vi "Two Button Dialog_TouchScreen.vi"(1 "F button name (\"Cancel\")":string, 2 "T button name (\"OK\")":string, 3 "Message":string) -> (0 "T Button?":T1)   [LabVIEW 2010]
uses:
  _TypeDefs/OK Button_TouchScreen.ctl
panel:
  in  "F Button":T1
  in  "T Button":T1
  out "Message Indicator":string
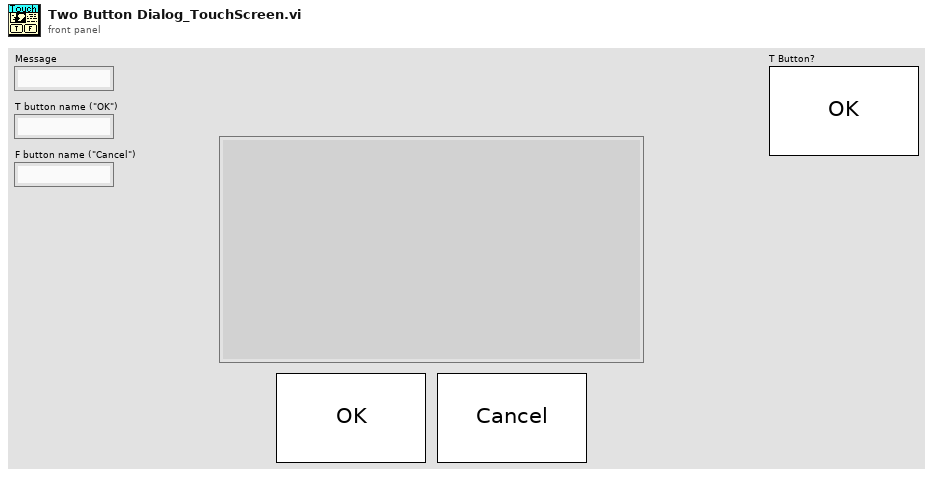
[diagram p1: front panel]
types:
  T1 = typedef "OK Button_TouchScreen.ctl" = bool
  T2 = enum8{"Enabled", "Disabled", "Disabled and Grayed Out"}
  T3 = cluster{"left":i16, "top":i16, "right":i16, "bottom":i16}
  T4 = typedef "LVBoundsTypeDef.ctl" = cluster{"Width":u32, "Height":u32}
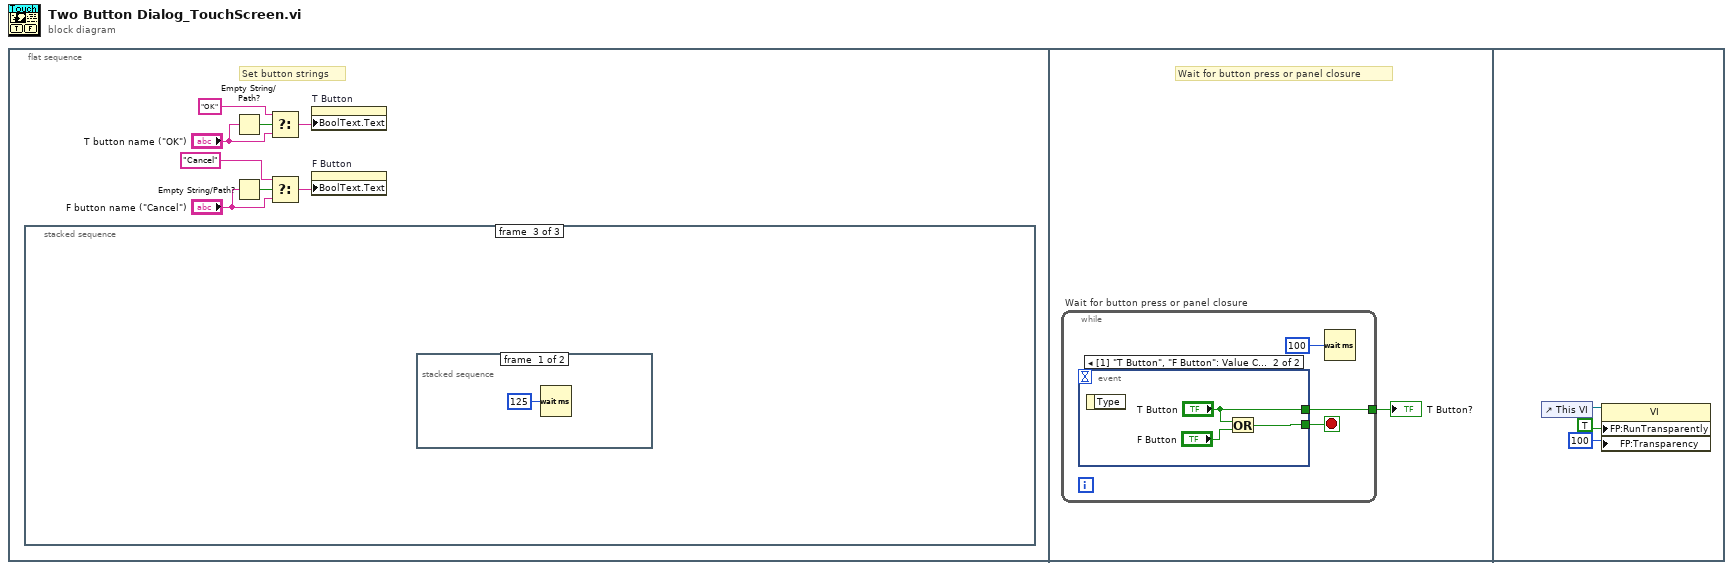
[diagram p0: block diagram]
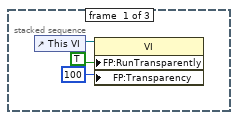
[diagram p2: hidden frame]
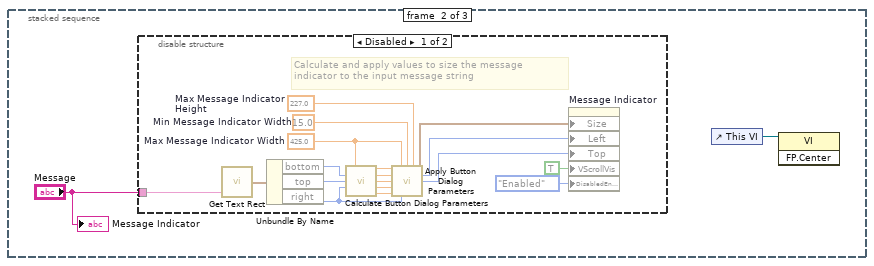
[diagram p3: hidden frame]
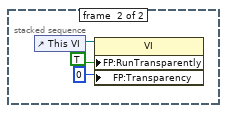
[diagram p5: hidden frame]
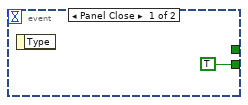
[diagram p6: hidden frame]
diagram:
  n1 = flat-sequence {
    frame #0 {
      # "Set button strings"
      n2 = stacked-sequence {
        frame #0 {
          n3 = control-ref of="This VI"() -> (w9:refnum<vi>)
          n4 = property class="VI"(reference=w9, "FP:RunTransparently"=TRUE, "FP:Transparency"=u8 100 ("Front Panel Window:Transparency")) -> ()  [unwired: 1 in, 2 out]
        }
        frame #1 {
          n5 = disable-structure shown="Disabled" {
            disable-tunnel: "Message" -> [w31 _]
            frame Disabled {
              w22 = 15.0  # Min Message Indicator Width
              w21 = 227.0  # Max Message Indicator Height
              w25 = 425.0  # Max Message Indicator Width
              # "Calculate and apply values to size the message indicator to the input message string"
              n6 = call <vilib>:"Get Text Rect.vi"("text"=w31) -> ("rect"=w29:T3)  [unwired: 8 in]
              n7 = Unbundle By Name(w29) -> ("bottom"=w17:i16, "top"=w18:i16, "right"=w16:i16)
              n8 = call "Calculate Button Dialog Parameters.vi"("Max Message Indicator Width"=w25, "bottom"=w17, "top"=w18, "right"=w16) -> ("Indicator left position"=w26:dbl, "Calculated indicator height"=w24:dbl, "Indicator height scaled large"=w23:dbl, "Actual indicator height"=w20:dbl, "Indicator height scaled small"=w19:dbl)  [unwired: 7 in]
              n9 = call "Apply Button Dialog Parameters.vi"("Indicator left position"=w26, "Max Message Indicator Width"=w25, "Min Message Indicator Width"=w22, "Max Message Indicator Height"=w21, "Calculated indicator height"=w24, "Indicator height scaled large"=w23, "Actual indicator height"=w20, "Indicator height scaled small"=w19, "right"=w16) -> ("Message indicator size"=w30:T4, "Message indicator left"=w28:i32, "Message indicator top"=w27:i32)  [unwired: 1 in, 3 out]
              n10 = property on="Message Indicator" class="Str"("Size"=w30, "Left"=w28, "Top"=w27, "VScrollVis"=TRUE ("Vertical Scrollbar Visible"), "DisabledEnum"=T2."Enabled" ("Disabled")) -> ()  [unwired: 2 in, 2 out]
            }
            frame Enabled {
            }
          }
          n11 = control-ref of="This VI"() -> (w12:refnum<vi>)
          n12 = invoke class="VI" method="FP.Center"(reference=w12) -> ()  [unwired: 2 in, 3 out]
          "Message Indicator" <- "Message"
        }
        frame #2 {
          n13 = stacked-sequence {
            frame #0 {
              n14 = Wait (ms)(milliseconds to wait=u32 125) -> ()  [unwired: 1 out]
            }
            frame #1 {
              n15 = control-ref of="This VI"() -> (w35:refnum<vi>)
              n16 = property class="VI"(reference=w35, "FP:RunTransparently"=TRUE, "FP:Transparency"=u8 0 ("Front Panel Window:Transparency")) -> ()  [unwired: 1 in, 2 out]
            }
          }
        }
      }
      n17 = Empty String/Path?(string/path="T button name (\"OK\")") -> (empty?=w7:bool)
      n18 = Empty String/Path?(string/path="F button name (\"Cancel\")") -> (empty?=w2:bool)
      n19 = Select(t="OK", s=w7, f="T button name (\"OK\")") -> (s? t:f=w5:string)
      n20 = Select(t="Cancel", s=w2, f="F button name (\"Cancel\")") -> (s? t:f=w1:string)
      n21 = property on="T Button" class="Bool"("BoolText.Text"=w5) -> ()  [unwired: 2 in, 2 out]
      n22 = property on="F Button" class="Bool"("BoolText.Text"=w1) -> ()  [unwired: 2 in, 2 out]
    }
    frame #1 {
      # "Wait for button press or panel closure"
      n23 = while "Wait for button press or panel closure" {
        tunnel: [w37] -> w36
        stop <- w38 stop-if-true
        n24 = event shown="[1] \"T Button\", \"F Button\": Value Change" {
          selector: _ -> [_ _]
          dyn-events: _ -> [_ _]
          timeout: _ -> [_ _]
          tunnel: [T1 TRUE ("T Button") w42] -> w38
          tunnel: [_ "T Button"] -> w37
          event Panel Close {
            n25 = event-data() -> ()  [unwired: 1 in, 1 out]
          }
          event Value Change {
            n26 = event-data() -> ()  [unwired: 1 in, 1 out]
            n27 = Or(x="T Button", y="F Button") -> (x .or. y?=w42:T1)
          }
        }
        n28 = Wait (ms)(milliseconds to wait=u32 100) -> ()  [unwired: 1 out]
      }
      "T Button?" <- w36
    }
    frame #2 {
      n29 = control-ref of="This VI"() -> (w46:refnum<vi>)
      n30 = property class="VI"(reference=w46, "FP:RunTransparently"=TRUE, "FP:Transparency"=u8 100 ("Front Panel Window:Transparency")) -> ()  [unwired: 1 in, 2 out]
    }
  }
